vi "ief_start_axis_absolut.vi"(3 "error in (no error)":errorcluster, 4 "Absolute Position":sgl format="%.2f", 5 "Axis Number":u16=1 min=1 max=16, 6 "Tagprefix in":refnum<k21>) -> (0 "error out (no error)":errorcluster, 1 "Start Position":sgl format="%.2f", 2 "Tagprefix out":refnum<k21>)   [LabVIEW 2015, in "IEF Werner.lvlib"]
doc: "The VI moves the chosen axis to the specified absolute position. Furthermore it returns the start position of the chosen axis before executing the start axis absolut command.\nUnlike the start manuell axis absolut command no supplemental control move axis command is needed.\n\nAxis Number Range:\n01, 10 hex\n1, 16 dec\n\nAbslute Position Range: 32 Bit Float"
uses:
  IEF Werner.lvlib
panel:
  # "IEF Start Axis Absolut"
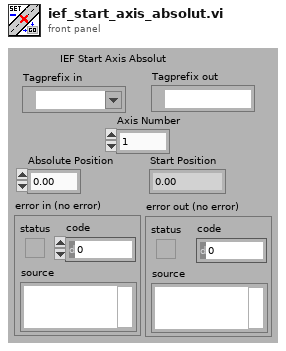
[diagram p1: front panel]
types:
  T1 = typedef "Semaphore RefNum" = refnum<k1>
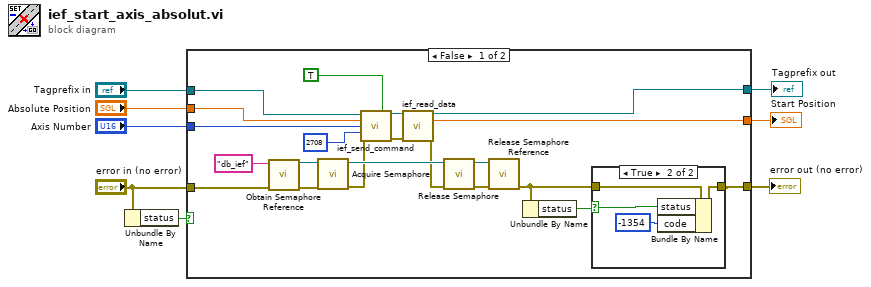
[diagram p0: block diagram]
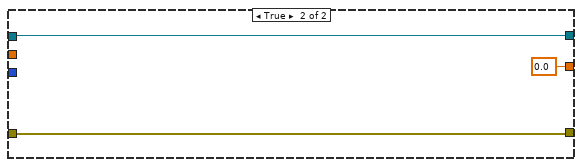
[diagram p3: hidden frame]
diagram:
  n1 = Unbundle By Name("error in (no error)") -> ("status"=w5:bool)
  n2 = case shown="False" w5 {
    tunnel: "Axis Number" -> [w22 _]
    tunnel: "Absolute Position" -> [w19 _]
    tunnel: "error in (no error)" -> [w17 w37]
    tunnel: [w16 w37] -> w4
    tunnel: [w12 sgl 0.0 ("value real 32")] -> w3
    tunnel: "Tagprefix in" -> [w11 w36]
    tunnel: [w9 w36] -> w1
    frame False {
      n3 = call <vilib>:"Obtain Semaphore Reference.vi"("error in (no error)"=w17, "name (unnamed)"="db_ief") -> ("error out"=w27:errorcluster, "semaphore"=w28:T1)  [unwired: 3 in, 1 out]
      n4 = call <vilib>:"Acquire Semaphore.vi"("error in (no error)"=w27, "semaphore"=w28) -> ("error out"=w25:errorcluster, "semaphore out"=w26:T1)  [unwired: 3 in, 1 out]
      n5 = call "ief_send_command.vi"("Tagprefix in"=w11, "Command datum of type real"=TRUE, "Command datum"=w19, "Command parameter"=w22, "Command code"=u16 2708, "error in (no error)"=w25) -> ("Tagprefix out"=w10:refnum<k21>, "error out (no error)"=w14:errorcluster)  [unwired: 4 in, 4 out]
      n6 = call "ief_read_data.vi"("Tagprefix in"=w10, "error in (no error)"=w14) -> ("Tagprefix out"=w9:refnum<k21>, "value real 32"=w12:sgl, "error out (no error)"=w13:errorcluster)  [unwired: 7 in, 4 out]
      n7 = call <vilib>:"Release Semaphore.vi"("error in (no error)"=w13, "semaphore"=w26) -> ("error out"=w24:errorcluster, "semaphore out"=w23:T1)  [unwired: 4 in]
      n8 = call <vilib>:"Release Semaphore Reference.vi"("error in (no error)"=w24, "semaphore"=w23) -> ("error out"=w15:errorcluster)  [unwired: 8 in, 1 out]
      n9 = Unbundle By Name(w15) -> ("status"=w18:bool)
      n10 = case shown="True" w18 {
        selector: w18 -> [_ w31]
        tunnel: [w30 w33] -> w16
        tunnel: w15 -> [w30 w34]
        frame False {
        }
        frame True {
          n11 = Bundle By Name(cluster=w34, "status"=w31, "code"=-1354) -> (w33:errorcluster)
        }
      }
    }
    frame True {
    }
  }
  "error out (no error)" <- w4
  "Start Position" <- w3
  "Tagprefix out" <- w1
